vi "Huber Test Program RS485.vi"() -> ()   [LabVIEW 2021, in "Huber Unistat 410 TCU.lvlib"]
uses:
  Huber Unistat 410 TCU.lvlib
  Huber Unistat 410 RS485 Settings.ctl
panel:
  out "Huber Unistat 410 Settings":T1 {"Address" min=0 max=99 format="%02.0f"}
  in  "Huber Unistat 410 Settings":T1 {"Address" min=0 max=99 format="%02.0f"}
  in  "Internal?":bool
  in  "Run":bool
  in  "Temp":dbl
  in  "stop":bool
  out "Connection Error":bool
  out "Running":bool
  out "Temperature":dbl
  out "error out":errorcluster
  in  "error in (no error)":errorcluster
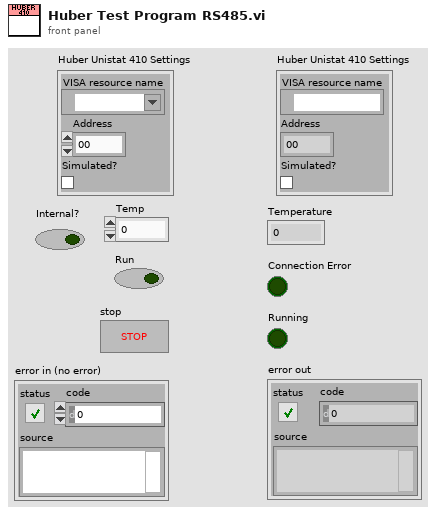
[diagram p1: front panel]
types:
  T1 = typedef "Huber Unistat 410 TCU.lvlib/Huber Unistat 410 RS485 Settings.ctl" = cluster{"VISA resource name":refnum<visa-resource-name>, "Address":i8, "Simulated?":bool}
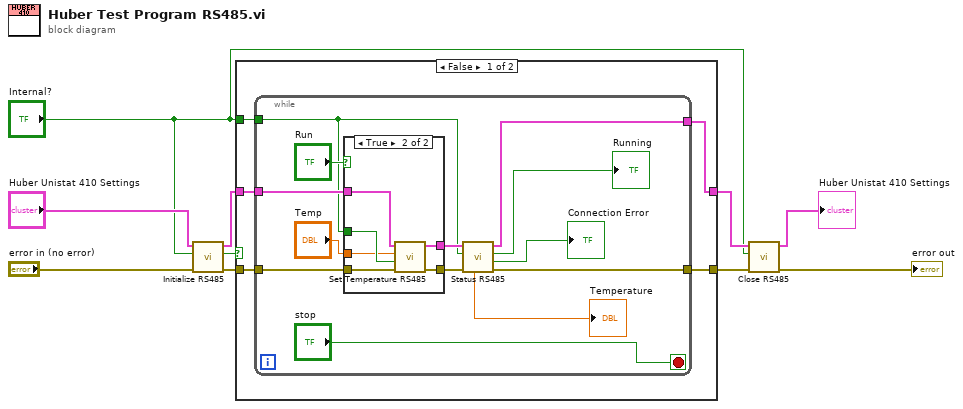
[diagram p0: block diagram]
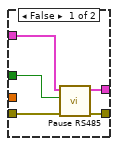
[diagram p2: hidden frame]
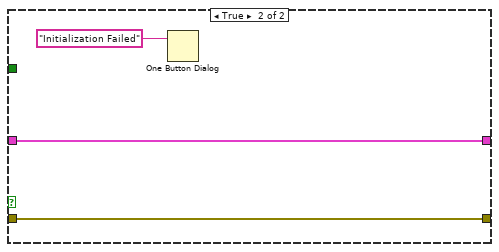
[diagram p3: hidden frame]
diagram:
  n1 = call "Initialize RS485.vi"("error in (no error)"="error in (no error)", "Internal?"="Internal?", "Huber Unistat 410 Settings"="Huber Unistat 410 Settings") -> ("error out"=w7:errorcluster, "Connection Error"=w6:bool, "Huber Unistat 410 Settings 2"=w8:T1)  [unwired: 6 in]
  n2 = case shown="False" w6 {
    tunnel: [w15 w41] -> w5
    tunnel: [w14 w40] -> w4
    tunnel: w8 -> [w13 w41]
    tunnel: w7 -> [w12 w40]
    tunnel: "Internal?" -> [w11 _]
    frame False {
      n3 = while {
        tunnel: [w16] -> w15
        tunnel: [w17] -> w14
        tunnel: w13 -> [w27]
        tunnel: w12 -> [w26]
        tunnel: w11 -> [w22]
        stop <- "stop" stop-if-true
        n4 = case shown="True" "Run" {
          tunnel: w27 -> [w33 w39]
          tunnel: w26 -> [w31 w36]
          tunnel: [w29 w34] -> w21
          tunnel: [w30 w35] -> w23
          tunnel: "Temp" -> [_ w37]
          tunnel: w22 -> [w32 w38]
          frame False {
            n5 = call "Pause RS485.vi"("error in (no error)"=w31, "Internal?"=w32, "Huber Unistat 410 Settings"=w33) -> ("error out"=w29:errorcluster, "Huber Unistat 410 Settings"=w30:T1)  [unwired: 7 in]
          }
          frame True {
            n6 = call "Set Temperature RS485.vi"("error in (no error)"=w36, "Internal?"=w38, "Setpoint"=w37, "Huber Unistat 410 Settings"=w39) -> ("error out"=w34:errorcluster, "Huber Unistat 410 Settings"=w35:T1)  [unwired: 5 in, 1 out]
          }
        }
        n7 = call "Status RS485.vi"("error in (no error)"=w21, "Internal?"=w22, "Huber Unistat 410 Settings"=w23) -> ("error out"=w17:errorcluster, "Connection Error"=→"Connection Error":bool, "Running"=→"Running":bool, "Huber Unistat 410 Settings"=w16:T1, "Temperature"=→"Temperature":dbl)  [unwired: 4 in]
      }
    }
    frame True {
      n8 = One Button Dialog(message="Initialization Failed") -> ()  [unwired: 1 in, 1 out]
    }
  }
  n9 = call "Close RS485.vi"("error in (no error)"=w4, "Internal?"="Internal?", "Huber Unistat 410 Settings"=w5) -> ("error out"=→"error out":errorcluster, "Huber Unistat 410 Settings"=→"Huber Unistat 410 Settings":T1)  [unwired: 7 in]
